vi "GetCurTimeStr.vi"() -> (0 "Time":string)   [LabVIEW 2016]
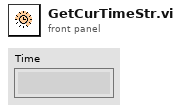
[diagram p1: front panel]
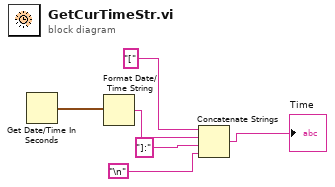
[diagram p0: block diagram]
diagram:
  n1 = Get Date/Time In Seconds() -> (seconds since 1Jan1904=w6:timestamp)
  n2 = Format Date/Time String(seconds (now)=w6) -> (date/time string=w4:string)  [unwired: 2 in]
  n3 = Concatenate Strings("[", w4, "]:" ("字符串"), "\n") -> (→"Time":string)
